vi "Close_Sim.vi"(11 "QuSim in":refnum<class "QuSim.lvclass">) -> (3 "QuSim out":refnum<class "QuSim.lvclass">)   [LabVIEW 2020, in "QuSim.lvclass"]
uses:
  QuSim.lvclass
  QuWire/QuWire.lvclass
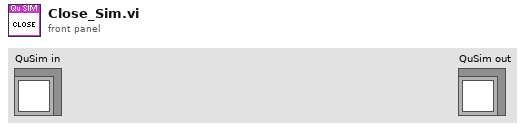
[diagram p1: front panel]
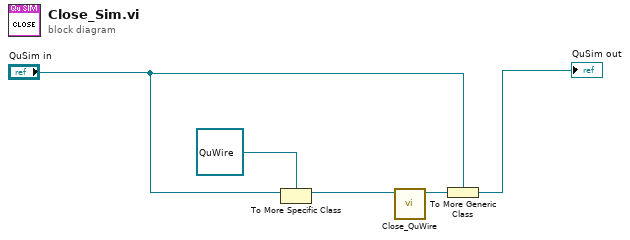
[diagram p0: block diagram]
diagram:
  n1 = To More Specific Class(target class=refnum<class "QuWire.lvclass"> refnum ("Wire.lvclass"), reference="QuSim in") -> (specific class reference=w1:refnum<class "QuWire.lvclass">)  [unwired: 1 in, 1 out]
  n2 = call "Close_QuWire.vi"("QuWire in"=w1) -> ("QuWire out"=w2:refnum<class "QuWire.lvclass">)  [unwired: 9 in, 1 out]
  n3 = To More Generic Class(target class="QuSim in", reference=w2) -> (generic class reference=→"QuSim out":refnum<class "QuSim.lvclass">)
